vi "sendLogMessage.vi"(8 "error in (no error)":errorcluster, 10 "message":string, 11 "tcpServer in":refnum<class "TcpServer.lvclass">) -> (0 "error out":errorcluster, 3 "tcpServer out":refnum<class "TcpServer.lvclass">)   [LabVIEW 2018]
doc: "Send a log message."
uses:
  src/TcpServer/TcpServer.lvclass
  src/TcpServerBase/typedef/connStatusCluster.ctl
  src/TcpServerCmd/TcpServerCmd.lvclass
  src/TcpServerBase/TcpServerBase.lvclass
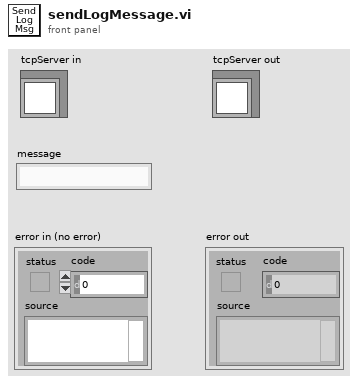
[diagram p1: front panel]
types:
  T1 = typedef "TcpServerBase.lvclass/connStatusCluster.ctl" = cluster{"connStatus":bool, "message":string}
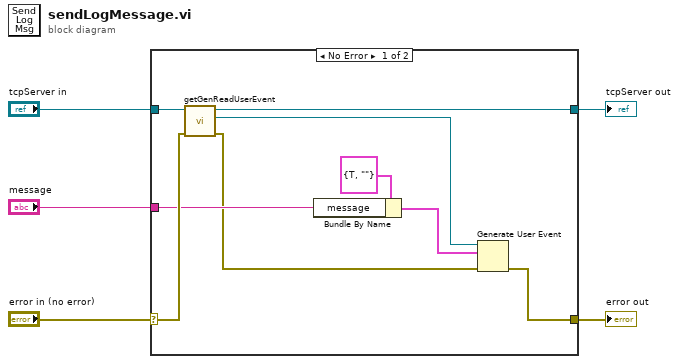
[diagram p0: block diagram]
diagram:
  n1 = case shown="No Error" "error in (no error)" {
    selector: "error in (no error)" -> [w12 w15]
    tunnel: "tcpServer in" -> [w14 w16]
    tunnel: [w13 w16] -> w4
    tunnel: "message" -> [w9 _]
    tunnel: [w8 w15] -> w1
    frame No Error {
      n2 = call "getGenReadUserEvent.vi"("error in (no error)"=w12, "TcpServer in"=w14) -> ("error out"=w7:errorcluster, "GenRead"=w11:refnum<user-event>, "TcpServer out"=w13:refnum<class "TcpServer.lvclass">)  [unwired: 7 in]
      n3 = Bundle By Name(cluster=T1 {"connStatus"=TRUE, "message"=""} ("t"), "message"=w9) -> (w6:T1)
      n4 = Generate User Event(user event=w11, event data cluster=w6, error in=w7) -> (error out=w8:errorcluster)  [unwired: 1 in, 1 out]
    }
    frame Error {
    }
  }
  "tcpServer out" <- w4
  "error out" <- w1
